vi "2 Tube Line Following.vi"(6 "Right Drive In":dbl, 8 "Left Drive In":dbl, 9 "Right Sensor":bool, 10 "Middle Sensor":bool, 11 "Left Sensor":bool) -> (1 "Right Drive Out":dbl, 2 "Left Drive Out":dbl)   [LabVIEW 2011]
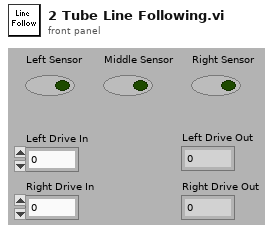
[diagram p1: front panel]
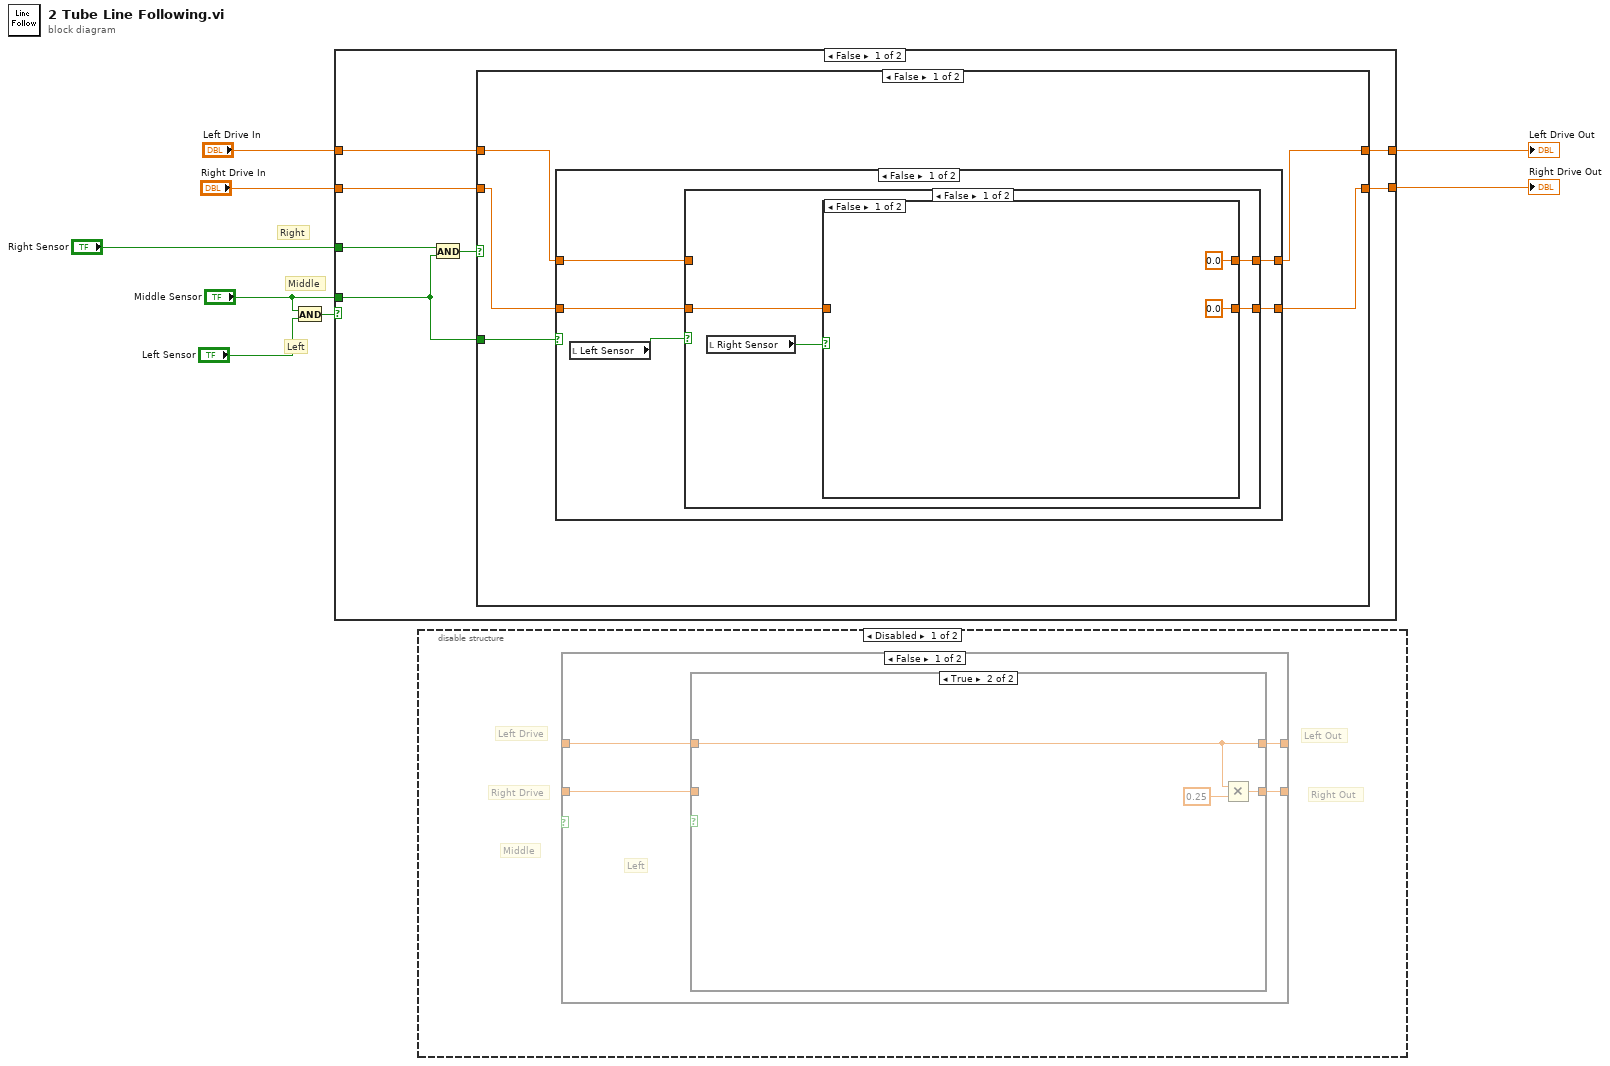
[diagram p0: block diagram]
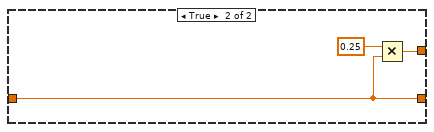
[diagram p2: hidden frame]
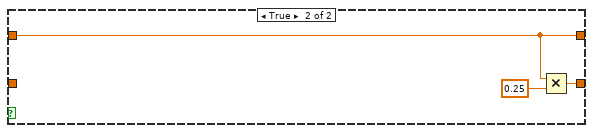
[diagram p3: hidden frame]
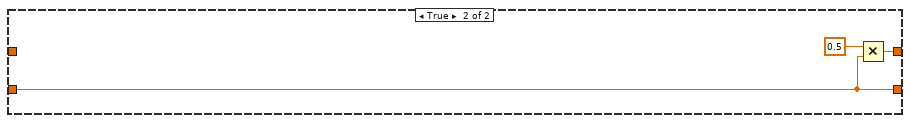
[diagram p5: hidden frame]
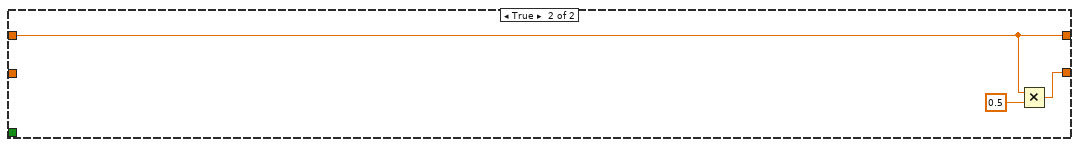
[diagram p6: hidden frame]
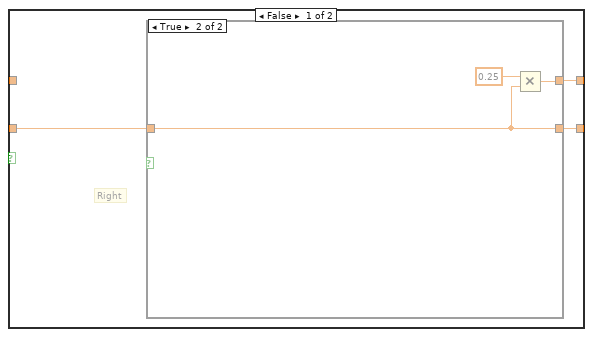
[diagram p7: hidden frame]
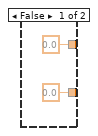
[diagram p8: hidden frame]
diagram:
  # "Right"
  # "Middle"
  # "Left"
  n1 = And(x="Middle Sensor", y="Left Sensor") -> (x .and. y?=w3:bool)
  n2 = case shown="False" w3 {
    tunnel: "Left Drive In" -> [w10 w45]
    tunnel: "Right Drive In" -> [w14 _]
    tunnel: [w12 w45] -> w5
    tunnel: [w13 w44] -> w4
    tunnel: "Middle Sensor" -> [w11 _]
    tunnel: "Right Sensor" -> [w9 _]
    frame False {
      n3 = And(x=w9, y=w11) -> (x .and. y?=w15:bool)
      n4 = case shown="False" w15 {
        tunnel: [w16 w41] -> w13
        tunnel: w14 -> [w18 w41]
        tunnel: [w17 w42] -> w12
        tunnel: w11 -> [w20 _]
        tunnel: w10 -> [w19 _]
        frame False {
          n5 = case shown="False" w20 {
            tunnel: w19 -> [w22 w39]
            tunnel: w18 -> [w25 w38]
            tunnel: [w23 w39] -> w17
            tunnel: [w24 w38] -> w16
            frame False {
              n6 = local read "Left Sensor"() -> (w21:bool)
              n7 = case shown="False" w21 {
                tunnel: [w29 w37] -> w24
                tunnel: w25 -> [w27 _]
                tunnel: [w28 w36] -> w23
                tunnel: w22 -> [_ w36]
                frame False {
                  n8 = local read "Right Sensor"() -> (w26:bool)
                  n9 = case shown="False" w26 {
                    tunnel: [0.0 w33] -> w29
                    tunnel: [0.0 ("Left Drive In") w34] -> w28
                    tunnel: w27 -> [_ w33]
                    frame False {
                    }
                    frame True {
                      n10 = Multiply(x=0.25, y=w33) -> (x*y=w34:dbl)
                    }
                  }
                }
                frame True {
                  n11 = Multiply(x=w36, y=0.25) -> (x*y=w37:dbl)
                }
              }
            }
            frame True {
            }
          }
        }
        frame True {
          n12 = Multiply(x=0.5, y=w41) -> (x*y=w42:dbl)
        }
      }
    }
    frame True {
      n13 = Multiply(x=w45, y=0.5) -> (x*y=w44:dbl)
    }
  }
  "Left Drive Out" <- w5
  "Right Drive Out" <- w4
  n14 = disable-structure shown="Disabled" {
    frame Disabled {
      # "Right Out"
      # "Left Out"
      # "Right Drive"
      # "Left Drive"
      # "Middle"
      n15 = case shown="False" {
        selector: _ -> [_ _]
        tunnel: _ -> [w46 w62]
        tunnel: _ -> [w49 w61]
        tunnel: [w47 w62] -> _
        tunnel: [w48 w61] -> _
        frame False {
          # "Left"
          n16 = case shown="True" {
            selector: _ -> [_ _]
            tunnel: [w52 w60] -> w48
            tunnel: w49 -> [w50 _]
            tunnel: [w51 w59] -> w47
            tunnel: w46 -> [_ w59]
            frame False {
              # "Right"
              n17 = case shown="True" {
                selector: _ -> [_ _]
                tunnel: [0.0 w56] -> w52
                tunnel: [0.0 ("Left Drive In") w57] -> w51
                tunnel: w50 -> [_ w56]
                frame False {
                }
                frame True {
                  n18 = Multiply(x=0.25, y=w56) -> (x*y=w57:dbl)
                }
              }
            }
            frame True {
              n19 = Multiply(x=w59, y=0.25) -> (x*y=w60:dbl)
            }
          }
        }
        frame True {
        }
      }
    }
    frame Enabled {
    }
  }
